vi "run_job.vi"(0 "REST Client in":refnum<class "REST Client.lvclass">, 1 "issue folder path":path, 3 "volume folder path":path, 5 "job queue":refnum<queue>, 9 "manager_daemon":refnum<class "manager_daemon.lvclass">, 11 "error in (no error)":errorcluster, 12 "files updated":string[](array[string])) -> (4 "REST Client out":refnum<class "REST Client.lvclass">, 6 "job queue out":refnum<queue>, 8 "Run Next":bool, 10 "status":string, 13 "job path":path, 14 "files updated out":string[](array[string]), 15 "error out":errorcluster)   [LabVIEW 2024, in "Download_Manager.lvlib"]
uses:
  Download_Manager.lvlib
  <vilib>/addons/_JKI.lib/REST Client/classes/REST Client/REST Client.lvclass
  typedefs/job--cluster.ctl
  typedefs/job_type--enum.ctl
  comic_manager/manager_daemon/manager_daemon.lvclass
  CV_RESTful_Library/typedefs/local_issue--cluster.ctl
  CV_RESTful_Library/typedefs/cv_issue.generic_credit--cluster.ctl
  CV_RESTful_Library/typedefs/cv_issue.associated_image--cluster.ctl
  CV_RESTful_Library/typedefs/cv_issue.person_credit--cluster.ctl
  CV_Shared_Library/volume.type--enum.ctl
  CV_RESTful_Library/CV_RESTful_Lib.lvlib
  <vilib>/addons/_JKI.lib/Serialization/JSON/JKI JSON Serialization.lvlib
  CV_Shared_Library/CV_Shared_Library.lvlib
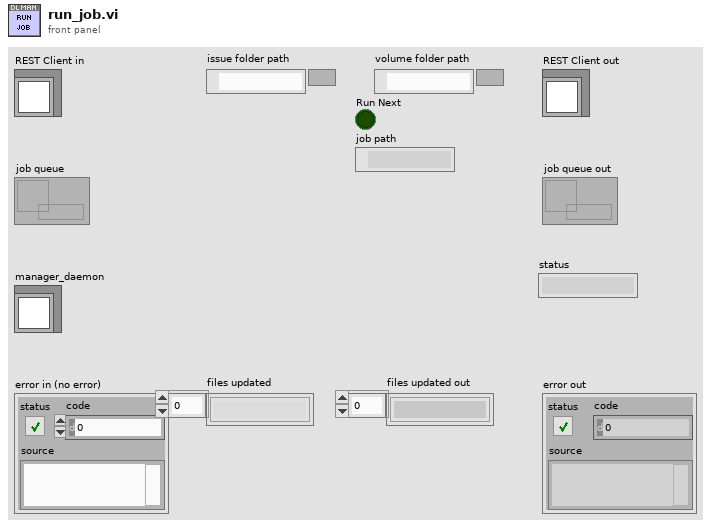
[diagram p1: front panel]
types:
  T1 = typedef "Download_Manager.lvlib/job--cluster.ctl" = cluster{"job type":T2, "job path":path, "id":i32, "url":string, "last updated":timestamp, "offset":i32, "original path":path}
  T2 = typedef "Download_Manager.lvlib/job_type--enum.ctl" = enum16{"check volume date", "check issues date", "download volume", "download isssue"}
  T3 = typedef "CV_Shared_Library.lvlib/volume.type--enum.ctl" = enum16{"Ongoing", "Limited Series", "Annual", "One Shot", "Reprint/Document", "Star Comics", "Epic Comics"}
  T4 = typedef "CV_RESTful_Lib.lvlib/cv_date_updated.results--array.ctl" = cluster{"date_last_updated":timestamp, "id":i32}[]
  T5 = typedef "CV_RESTful_Lib.lvlib/local_issue--cluster.ctl" = cluster{"cover_date":timestamp, "id":i32, "cv_id":string, "name":string, "sortable_name":string, "issue_number":string, "deck":string, "description":string, "volume":T6, "store_date":timestamp, "date_last_updated":timestamp, "site_detail_url":string, "cover_url":string, "associated_images":T7[], "characters":T6[], "concepts":T6[], "creators":T8[], "storyArcs":T6[], "teams":T6[]}
  T6 = typedef "CV_RESTful_Lib.lvlib/cv_issue.generic_credit--cluster.ctl" = cluster{"id":i32, "name":string}
  T7 = typedef "CV_RESTful_Lib.lvlib/cv_issue.associated_image--cluster.ctl" = cluster{"original_url":string, "id":i32}
  T8 = typedef "CV_RESTful_Lib.lvlib/cv_issue.person_credit--cluster.ctl" = cluster{"id":i32, "name":string, "role":string}
  T9 = typedef "CV_RESTful_Lib.lvlib/local_volume--cluster.ctl" = cluster{"id":i32, "name":string, "sortable_name":string, "aliases":string[], "description":string, "site_detail_url":string, "count_of_issues":i32, "start_year":i32, "publisher_id":i32, "issue_ids":i32[], "date_last_updated":timestamp, "volume":i32, "cv_id":string, "volume type":T3}
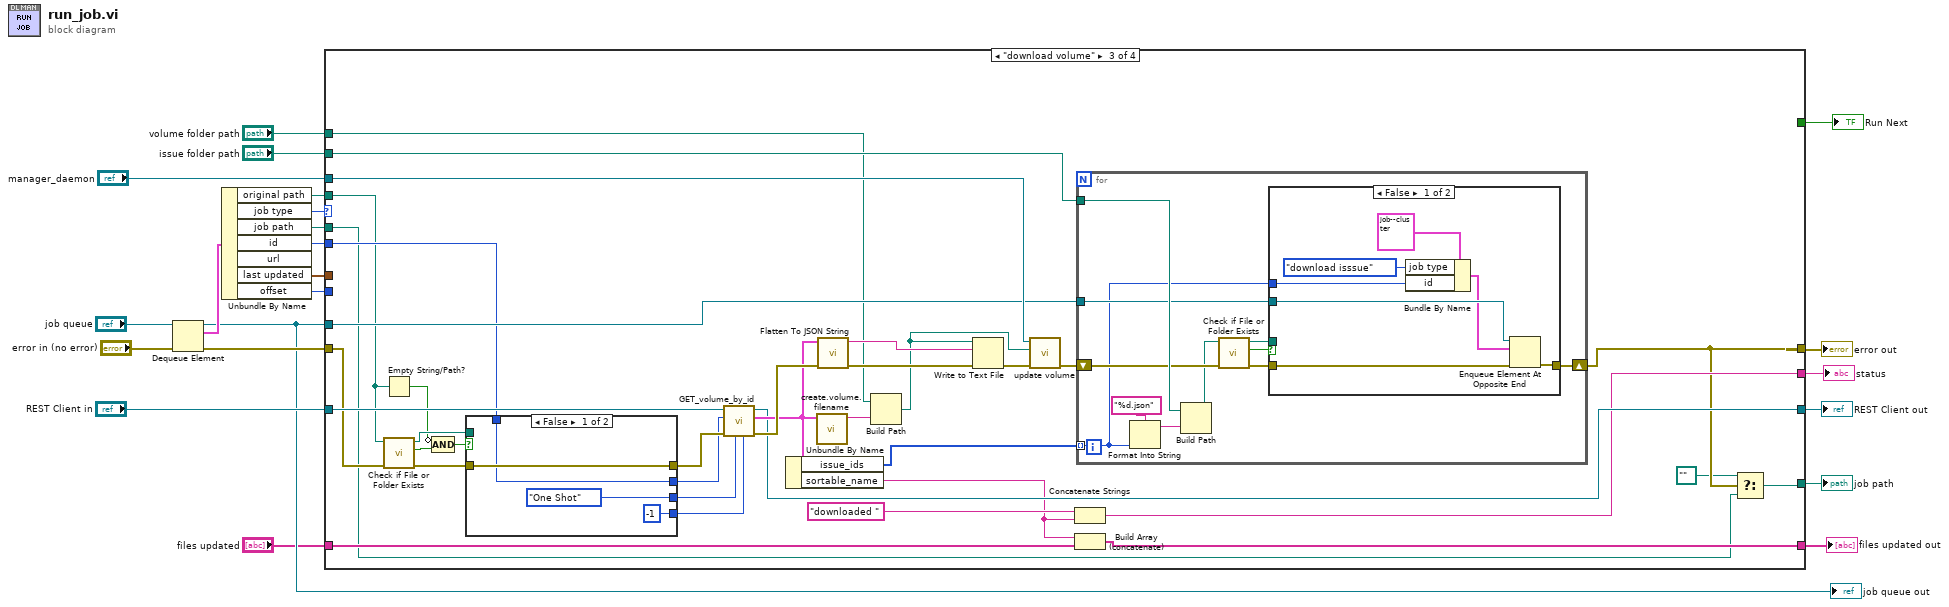
[diagram p0: block diagram]
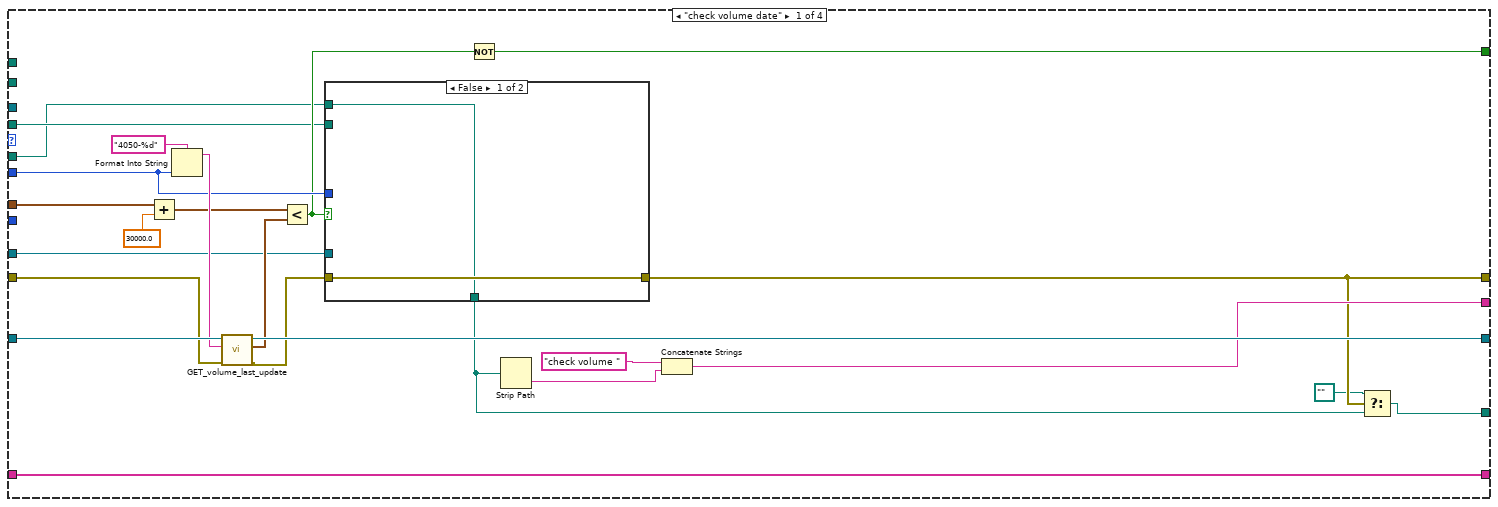
[diagram p2: hidden frame]
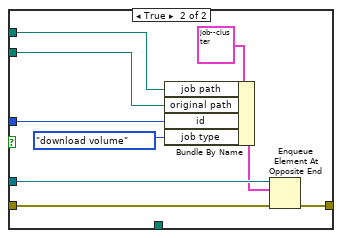
[diagram p3: hidden frame]
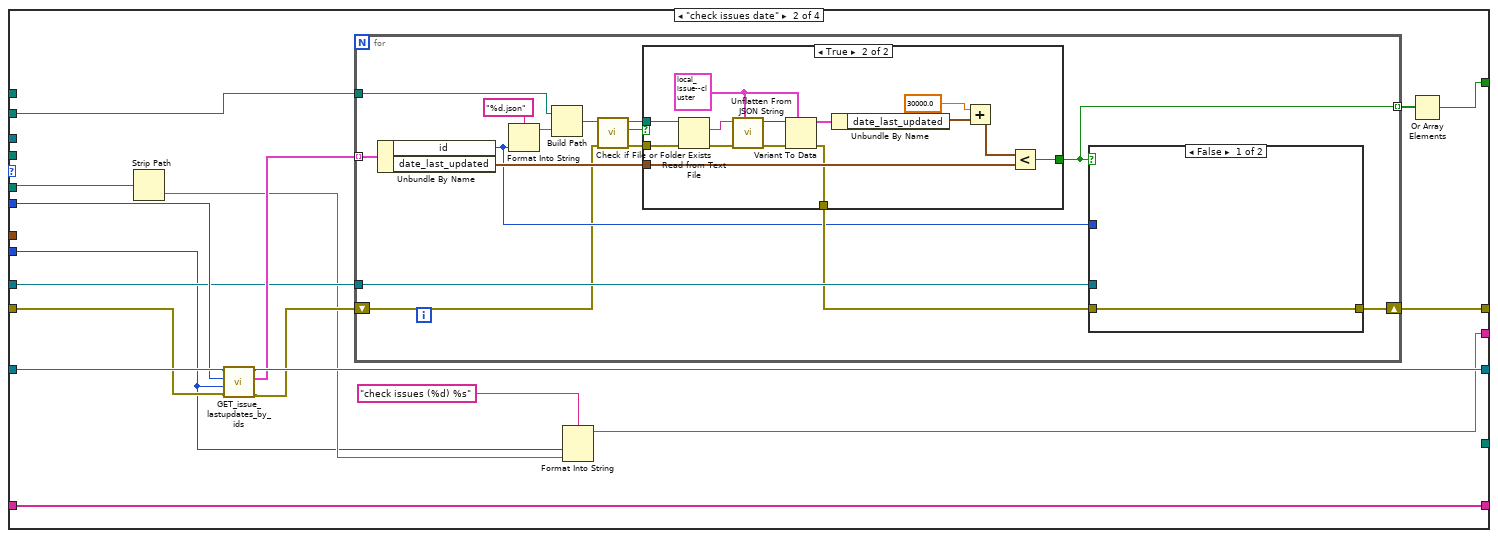
[diagram p4: hidden frame]
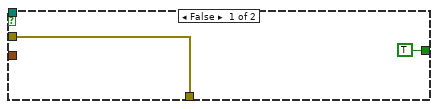
[diagram p5: hidden frame]
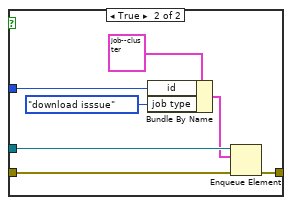
[diagram p6: hidden frame]
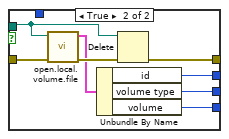
[diagram p7: hidden frame]
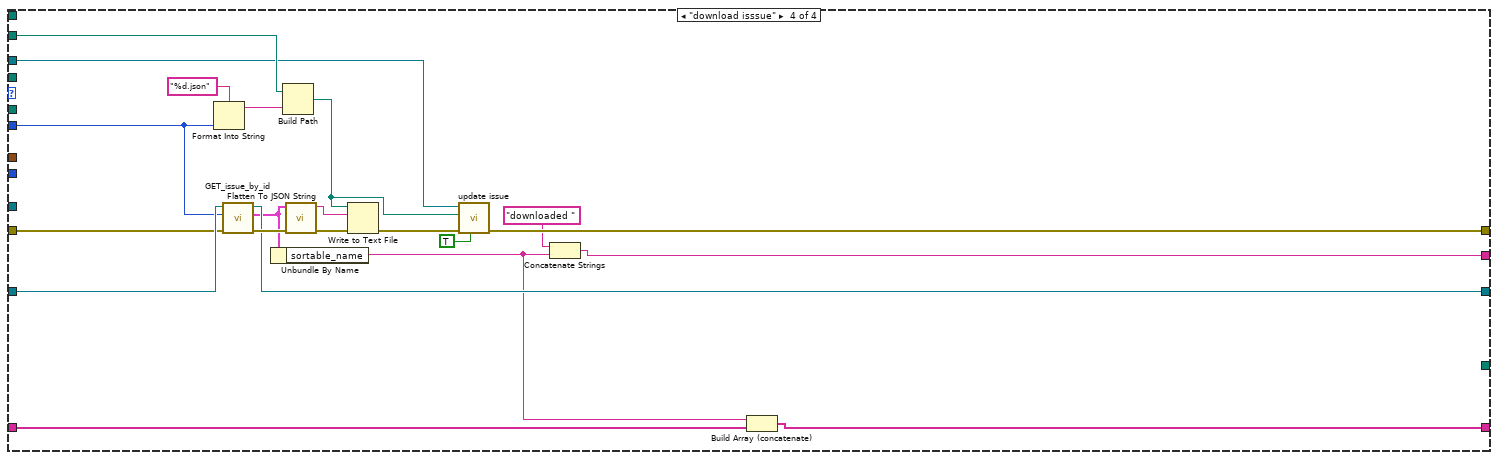
[diagram p9: hidden frame]
diagram:
  n1 = Dequeue Element(queue="job queue", error in (no error)="error in (no error)") -> (queue out=w8:refnum<queue>, element=w21:T1, error out=w17:errorcluster)  [unwired: 1 in, 1 out]
  "job queue out" <- w8
  n2 = Unbundle By Name(w21) -> ("original path"=w2:path, "job type"=w20:T2, "job path"=w10:path, "id"=w16:i32, "last updated"=w15:timestamp, "offset"=w6:i32)  [unwired: 1 out]
  n3 = case shown="\"download volume\"" w20 {
    tunnel: "REST Client in" -> [w46 w74 w135 w196]
    tunnel: w17 -> [w45 w71 w122 w194]
    tunnel: w16 -> [w35 w72 w125 w191]
    tunnel: [w42 w73 w132 w195] -> w12
    tunnel: w15 -> [w41 _ _ _]
    tunnel: w8 -> [w37 w68 w133 _]
    tunnel: [w26 w66 w117 w193] -> w13
    tunnel: "issue folder path" -> [_ w69 w134 w189]
    tunnel: "manager_daemon" -> [_ _ w136 w188]
    tunnel: w10 -> [w27 w65 w116 _]
    tunnel: "volume folder path" -> [_ _ w126 _]
    tunnel: [w32 w62 w130 w185] -> w7
    tunnel: w6 -> [_ w60 _ _]
    tunnel: "files updated" -> [w31 w64 w129 w183]
    tunnel: [w31 w64 w127 w182] -> w4
    tunnel: [w29 w58 _ _] -> w3
    tunnel: w2 -> [w28 _ w118 _]
    tunnel: [w24 _ w115 _] -> w1
    frame "check volume date" {
      n4 = Add(x=w41, y=30000.0) -> (x+y=w39:timestamp)
      n5 = Format Into String(format string="4050-%d", w35) -> (resulting string=w43:string)  [unwired: 2 in, 1 out]
      n6 = call "GET_volume_last_update.vi"("error in (no error)"=w45, "volume id"=w43, "REST Client in"=w46) -> ("error out"=w36:errorcluster, "results.date_last_updated"=w38:timestamp, "REST Client out"=w42:refnum<class "REST Client.lvclass">)  [unwired: 6 in]
      n7 = Less?(x=w39, y=w38) -> (x < y?=w30:bool)
      n8 = case shown="False" w30 {
        tunnel: w37 -> [_ w57]
        tunnel: w36 -> [w48 w56]
        tunnel: w35 -> [_ w54]
        tunnel: [w48 w51] -> w26
        tunnel: w28 -> [_ w50]
        tunnel: [w47 _] -> w25
        tunnel: w27 -> [w47 w49]
        frame False {
        }
        frame True {
          n9 = Bundle By Name(cluster=T1 {"job type"=enum."check volume date", "job path"=path "", "id"=0, "url"="", "last updated"=timestamp(0 s since 1904-01-01), "offset"=0, "original path"=path ""} ("element"), "job path"=w49, "original path"=w50, "id"=w54, "job type"=job_type--enum."download volume") -> (w52:T1)
          n10 = Enqueue Element At Opposite End(queue=w57, element=w52, error in (no error)=w56) -> (error out=w51:errorcluster)  [unwired: 1 in, 2 out]
        }
      }
      n11 = Not(x=w30) -> (.not. x?=w29:bool)
      n12 = Strip Path(path=w25) -> (name=w33:string)  [unwired: 1 out]
      n13 = Concatenate Strings("check volume ", w33) -> (w32:string)
      n14 = Select(t=path "", s=w26, f=w25) -> (s? t:f=w24:path)
    }
    frame "check issues date" {
      n15 = Strip Path(path=w65) -> (name=w61:string)  [unwired: 1 out]
      n16 = call "GET_issue_lastupdates_by_ids.vi"("error in (no error)"=w71, "offset"=w60, "volume id"=w72, "REST Client in"=w74) -> ("error out"=w67:errorcluster, "results"=w70:T4, "REST Client out"=w73:refnum<class "REST Client.lvclass">)  [unwired: 5 in]
      n17 = for {
        tunnel: w70 -> [w89] mode=indexing
        tunnel: w69 -> [w86]
        tunnel: w68 -> [w84]
        shift-right: [w81] -> w66
        shift-left: w67 -> [w76]
        tunnel: [w80] -> w59 mode=indexing
        n18 = Unbundle By Name(w89) -> ("id"=w82:i32, "date_last_updated"=w85:timestamp)
        n19 = Format Into String(format string="%d.json", w82) -> (resulting string=w87:string)  [unwired: 2 in, 1 out]
        n20 = Build Path(base path=w86, name or relative path=w87) -> (appended path=w79:path)
        n21 = call <vilib>:"Check if File or Folder Exists.vi"("error in (no error)"=w76, "path"=w79) -> ("error out"=w75:errorcluster, "file or folder exists?"=w77:bool, "dup path"=w78:path)  [unwired: 7 in]
        n22 = case shown="True" w77 {
          tunnel: w78 -> [_ w105]
          tunnel: w85 -> [_ w95]
          tunnel: [w90 w94] -> w83
          tunnel: [TRUE w93] -> w80
          tunnel: w75 -> [w90 w92]
          frame False {
          }
          frame True {
            w100 = T5 {"cover_date"=timestamp(0 s since 1904-01-01), "id"=0, "cv_id"="", "name"="", "sortable_name"="", "issue_number"="", "deck"="", "description"="", "volume"={"id"=0, "name"=""}, "store_date"=timestamp(0 s since 1904-01-01), "date_last_updated"=timestamp(0 s since 1904-01-01), "site_detail_url"="", "cover_url"="", "associated_images"=[], "characters"=[], "concepts"=[], "creators"=[], "storyArcs"=[], "teams"=[]} ("issue")
            n23 = Read from Text File(file (use dialog)=w105, error in=w92) -> (text=w103:string, error out=w104:errorcluster)  [unwired: 2 in, 2 out]
            n24 = call <vilib>:"Unflatten From JSON String.vi"("Type and Defaults"=w100, "error in"=w104, "JSON String"=w103) -> ("error out"=w102:errorcluster, "Variant"=w101:variant)  [unwired: 7 in]
            n25 = Variant To Data(error in=w102, type=w100, Variant=w101) -> (data=w99:T5, error out=w94:errorcluster)
            n26 = Unbundle By Name(w99) -> ("date_last_updated"=w98:timestamp)
            n27 = Add(x=30000.0, y=w98) -> (x+y=w96:timestamp)
            n28 = Less?(x=w96, y=w95) -> (x < y?=w93:bool)
          }
        }
        n29 = case shown="False" w80 {
          tunnel: w84 -> [_ w113]
          tunnel: w83 -> [w106 w112]
          tunnel: w82 -> [_ w110]
          tunnel: [w106 w107] -> w81
          frame False {
          }
          frame True {
            n30 = Bundle By Name(cluster=T1 {"job type"=enum."check volume date", "job path"=path "", "id"=0, "url"="", "last updated"=timestamp(0 s since 1904-01-01), "offset"=0, "original path"=path ""} ("element"), "id"=w110, "job type"=job_type--enum."download isssue") -> (w108:T1)
            n31 = Enqueue Element(queue=w113, element=w108, error in (no error)=w112) -> (error out=w107:errorcluster)  [unwired: 1 in, 2 out]
          }
        }
      }
      n32 = Format Into String(format string="check issues (%d) %s", w60, w61) -> (resulting string=w62:string)  [unwired: 2 in, 1 out]
      n33 = Or Array Elements(Boolean array=w59) -> (logical OR=w58:bool)
    }
    frame "download volume" {
      n34 = Empty String/Path?(string/path=w118) -> (empty?=w119:bool)
      n35 = call <vilib>:"Check if File or Folder Exists.vi"("error in (no error)"=w122, "path"=w118) -> ("error out"=w123:errorcluster, "file or folder exists?"=w120:bool, "dup path"=w124:path)  [unwired: 7 in]
      n36 = Compound Arithmetic op=AND(invert w119, w120) -> (w121:bool)
      n37 = case shown="False" w121 {
        tunnel: [volume.type--enum."One Shot" ("volume type") w161] -> w143
        tunnel: [w153 w160] -> w142
        tunnel: [w152 w159] -> w141
        tunnel: [-1 ("volume") w158] -> w137
        tunnel: w123 -> [w153 w157]
        tunnel: w124 -> [_ w154]
        tunnel: w125 -> [w152 _]
        frame False {
        }
        frame True {
          n38 = call "open.local.volume.file.vi"("error in (no error)"=w157, "volume json"=w154) -> ("error out"=w156:errorcluster, "volume"=w155:T9)  [unwired: 8 in]
          n39 = Unbundle By Name(w155) -> ("id"=w159:i32, "volume type"=w161:T3, "volume"=w158:i32)
          n40 = Delete(path (use dialog)=w154, error in=w156) -> (error out=w160:errorcluster)  [unwired: 3 in, 2 out]
        }
      }
      n41 = call "GET_volume_by_id.vi"("volume"=w137, "volume type"=w143, "error in (no error)"=w142, "volume id"=w141, "REST Client in"=w135) -> ("error out"=w148:errorcluster, "local volume"=w145:T9, "REST Client out"=w132:refnum<class "REST Client.lvclass">)  [unwired: 4 in]
      n42 = Unbundle By Name(w145) -> ("issue_ids"=w144:i32[], "sortable_name"=w128:string)
      n43 = call "create.volume.filename.vi"("volume"=w145) -> ("json filename"=w149:string)  [unwired: 10 in]
      n44 = call <vilib>:"Flatten To JSON String.vi"("error in"=w148, "Variant"=w145) -> ("error out"=w146:errorcluster, "JSON String"=w147:string)  [unwired: 8 in]
      n45 = Build Path(base path=w126, name or relative path=w149) -> (appended path=w138:path)
      n46 = Write to Text File(file (use dialog)=w138, text=w147, error in=w146) -> (error out=w140:errorcluster)  [unwired: 1 in, 2 out]
      n47 = call "update volume.vi"("error in (no error)"=w140, "Volume Path"=w138, "manager_daemon in"=w136) -> ("error out"=w139:errorcluster)  [unwired: 7 in, 1 out]
      n48 = Concatenate Strings("downloaded ", w128) -> (w130:string)
      n49 = Build Array (concatenate)(w128, w129) -> (w127:string[])
      n50 = for {
        tunnel: w144 -> [w162] mode=indexing
        tunnel: w134 -> [w170]
        shift-right: [w165] -> w117
        shift-left: w139 -> [w169]
        tunnel: w133 -> [w164]
        n51 = Format Into String(format string="%d.json", w162) -> (resulting string=w171:string)  [unwired: 2 in, 1 out]
        n52 = Build Path(base path=w170, name or relative path=w171) -> (appended path=w168:path)
        n53 = call <vilib>:"Check if File or Folder Exists.vi"("error in (no error)"=w169, "path"=w168) -> ("error out"=w166:errorcluster, "file or folder exists?"=w167:bool, "dup path"=w163:path)  [unwired: 7 in]
        n54 = case shown="False" w167 {
          tunnel: w166 -> [w179 w180]
          tunnel: [w177 w180] -> w165
          tunnel: w164 -> [w178 _]
          tunnel: w163 -> [_ _]
          tunnel: w162 -> [w173 _]
          frame False {
            n55 = Bundle By Name(cluster=T1 {"job type"=enum."check volume date", "job path"=path "", "id"=0, "url"="", "last updated"=timestamp(0 s since 1904-01-01), "offset"=0, "original path"=path ""} ("element"), "job type"=job_type--enum."download isssue", "id"=w173) -> (w174:T1)
            n56 = Enqueue Element At Opposite End(queue=w178, element=w174, error in (no error)=w179) -> (error out=w177:errorcluster)  [unwired: 1 in, 2 out]
          }
          frame True {
          }
        }
      }
      n57 = Select(t=path "", s=w117, f=w116) -> (s? t:f=w115:path)
    }
    frame "download isssue" {
      n58 = Format Into String(format string="%d.json", w191) -> (resulting string=w190:string)  [unwired: 2 in, 1 out]
      n59 = call "GET_issue_by_id.vi"("error in (no error)"=w194, "issue id"=w191, "REST Client in"=w196) -> ("error out"=w201:errorcluster, "local_issue"=w187:T5, "REST Client out"=w195:refnum<class "REST Client.lvclass">)  [unwired: 6 in]
      n60 = Unbundle By Name(w187) -> ("sortable_name"=w184:string)
      n61 = Build Path(base path=w189, name or relative path=w190) -> (appended path=w181:path)
      n62 = call <vilib>:"Flatten To JSON String.vi"("error in"=w201, "Variant"=w187) -> ("error out"=w200:errorcluster, "JSON String"=w199:string)  [unwired: 8 in]
      n63 = Write to Text File(file (use dialog)=w181, text=w199, error in=w200) -> (error out=w198:errorcluster)  [unwired: 1 in, 2 out]
      n64 = call "update issue.vi"("Update All (T)"=TRUE, "error in (no error)"=w198, "Issue Path"=w181, "manager_daemon in"=w188) -> ("error out"=w193:errorcluster)  [unwired: 6 in, 1 out]
      n65 = Concatenate Strings("downloaded ", w184) -> (w185:string)
      n66 = Build Array (concatenate)(w184, w183) -> (w182:string[])
    }
  }
  "error out" <- w13
  "REST Client out" <- w12
  "status" <- w7
  "files updated out" <- w4
  "Run Next" <- w3
  "job path" <- w1
